vi "new report subVI.vi"(0 "report in":refnum<class "ooWriter.lvclass">, 1 "window state (normal)":T1(ring)=enum."normal", 5 "display alerts? (F)":bool, 7 "template (empty)":path, 9 "machine name (empty)":string, 11 "error in (no error)":errorcluster) -> (4 "report out":refnum<class "ooWriter.lvclass">, 15 "error out":errorcluster)   [LabVIEW 2009, in "ooWriter.lvclass"]
uses:
  ooWriter.lvclass
  <vilib>/Utility/NIReport.llb/NI_report.lvclass
  C:/Projets/LAVAG/OpenOfficeRGT/AODL/DLLs/AODL.dll
  ooWriter.lvclass/ooWriter.ctl
  <vilib>/Utility/NIReport.llb/NI_ReportGenerationCore.lvlib
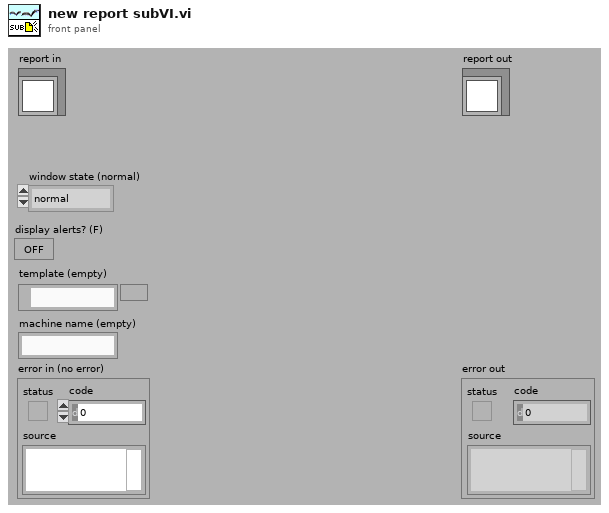
[diagram p1: front panel]
types:
  T1 = enum16{"maximized", "minimized", "normal", "no change"}
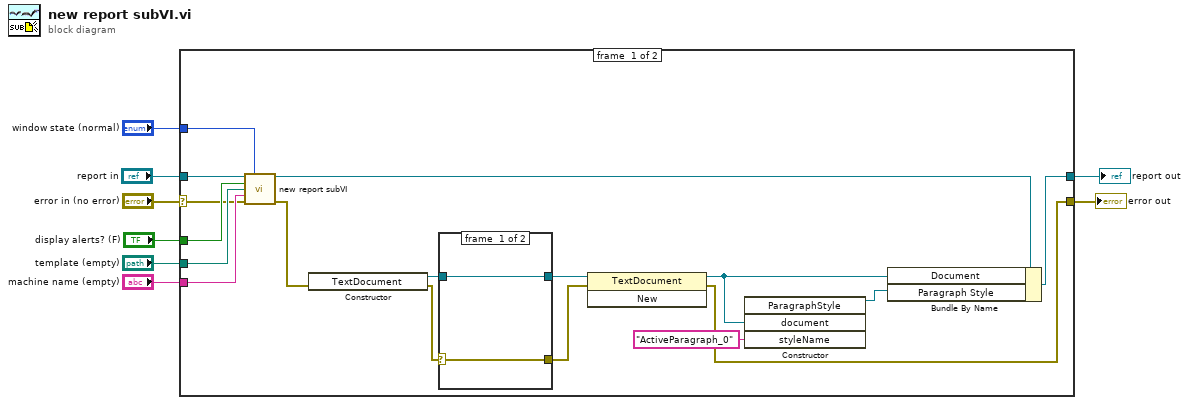
[diagram p0: block diagram]
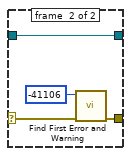
[diagram p2: hidden frame]
diagram:
  n1 = case shown="No Error" "error in (no error)" {
    selector: "error in (no error)" -> [w20 w32]
    tunnel: "report in" -> [w25 w33]
    tunnel: "window state (normal)" -> [w24 _]
    tunnel: [w18 w33] -> w6
    tunnel: "template (empty)" -> [w23 _]
    tunnel: "machine name (empty)" -> [w22 _]
    tunnel: [w13 w32] -> w3
    tunnel: "display alerts? (F)" -> [w21 _]
    frame #0 {
      n2 = call-parent "new report subVI.vi"("report in"=w25, "window state (normal)"=w24, "display alerts? (F)"=w21, "template (empty)"=w23, "machine name (empty)"=w22, "error in (no error)"=w20) -> ("report out"=w19:refnum<class "ooWriter.lvclass">, "error out"=w17:errorcluster)  [unwired: 8 in]
      n3 = constructor class="TextDocument"(error in=w17) -> (reference out=w15:refnum<k24>, error out=w16:errorcluster)  [unwired: 2 in, 1 out]
      n4 = case shown="Error" w16 {
        selector: w16 -> [w27 w29]
        tunnel: [w27 w30] -> w12
        tunnel: [w26 w28] -> w14
        tunnel: w15 -> [w26 w28]
        frame #0 {
        }
        frame #1 {
          n5 = call <vilib>:"Find First Error and Warning.vi"("error in (no error)"=w29, "error code"=-41106) -> ("error out"=w30:errorcluster)  [unwired: 5 out]
        }
      }
      n6 = invoke class="TextDocument" method="New"(reference=w14, error in=w12) -> (reference out=w11:refnum<k24>, error out=w13:errorcluster)  [unwired: 1 in, 1 out]
      n7 = constructor class="ParagraphStyle"("document"=w11, "styleName"="ActiveParagraph_0") -> (reference out=w9:refnum<k24>)  [unwired: 3 in, 4 out]
      n8 = Bundle By Name(cluster=w19, "Document"=w11, "Paragraph Style"=w9) -> (w18:refnum<class "ooWriter.lvclass">)
    }
    frame #1 {
    }
  }
  "error out" <- w3
  "report out" <- w6
